vi "arrows整体图.vi"() -> ()   [LabVIEW 2014]
panel:
  in  "Down 3":bool
  in  "Up 3":bool
  in  "Right 2":bool
  in  "Left 2":bool
  in  "Down 2":bool
  in  "Up 2":bool
  in  "Right":bool
  in  "Left":bool
  in  "Develop":bool
  in  "Bottom":bool
  in  "Back":bool
  in  "Up":bool
  in  "Undo":bool
  in  "Top":bool
  in  "Start":bool
  in  "Reload":bool
  in  "Redo":bool
  in  "Previous":bool
  in  "Next":bool
  in  "Loop":bool
  in  "Forward":bool
  in  "Finish":bool
  in  "Down":bool
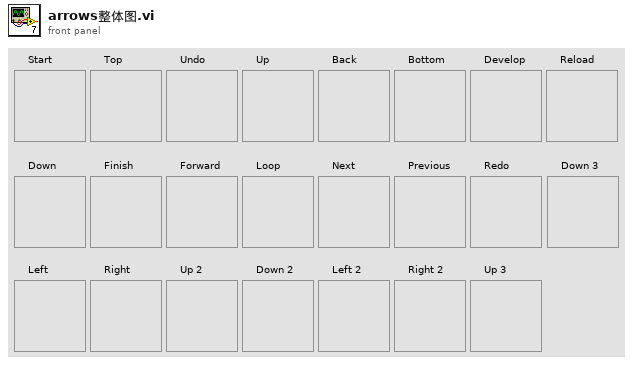
[diagram p1: front panel]
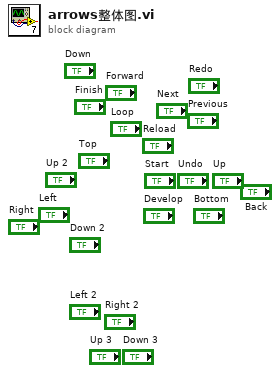
[diagram p0: block diagram]
diagram:
